vi "Accept Multiple.vi"(8 "error in (no error)":errorcluster, 9 "Number":i32, 10 "Accepted Runes":string, 11 "JSON Lexer in":refnum<class "JSON Lexer.lvclass">) -> (0 "error out":errorcluster, 1 "EOF":bool, 2 "Accepted?":bool, 3 "JSON Lexer out":refnum<class "JSON Lexer.lvclass">)   [LabVIEW 2013, in "JKI JSON Serialization.lvlib" / "JSON Lexer.lvclass"]
uses:
  JSON Lexer.lvclass
  JSON Lexer.lvclass/JSON Lexer.ctl
  <vilib>/addons/_JKI.lib/Unicode/UTF-8 String/UTF-8 String.lvclass/UTF-8 String.ctl
  <vilib>/addons/_JKI.lib/Unicode/UTF-8 String/Index Rune as UTF-8 Substring.vi
  <vilib>/addons/_JKI.lib/Unicode/UTF-8 String/Next Rune As UTF-8 Substring.vi
  <vilib>/addons/_JKI.lib/Unicode/UTF-8 String/Bytes In Rune.vi
  <vilib>/Utility/error.llb/Error Cluster From Error Code.vi
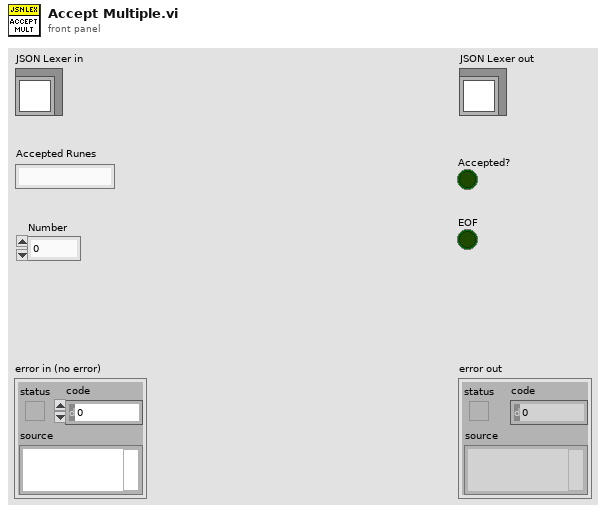
[diagram p1: front panel]
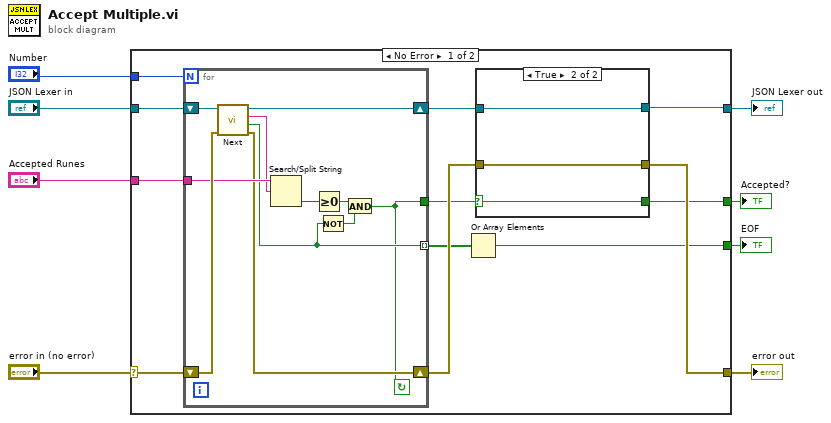
[diagram p0: block diagram]
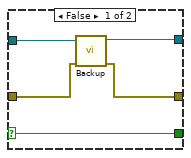
[diagram p2: hidden frame]
diagram:
  n1 = case shown="No Error" "error in (no error)" {
    selector: "error in (no error)" -> [w19 w41]
    tunnel: [w16 w41] -> w7
    tunnel: [w14 w40] -> w5
    tunnel: "JSON Lexer in" -> [w20 w40]
    tunnel: "Accepted Runes" -> [w18 _]
    tunnel: "Number" -> [w13 _]
    tunnel: [w10 _] -> w2
    tunnel: [w9 _] -> w1
    frame No Error {
      n2 = for {
        N: w13 -> [_]
        tunnel: w18 -> [w37]
        shift-right: [w33] -> w15
        shift-left: w20 -> [w39]
        shift-right: [w34] -> w17
        shift-left: w19 -> [w38]
        tunnel: [w29] -> w12
        tunnel: [w30] -> w11 mode=indexing
        stop <- w29 continue-if-true
        n3 = call "Next.vi"("error in (no error)"=w38, "JSON Lexer in"=w39) -> ("error out"=w34:errorcluster, "EOF"=w30:bool, "Rune"=w36:string, "JSON Lexer out"=w33:refnum<class "JSON Lexer.lvclass">)  [unwired: 6 in]
        n4 = Search/Split String(string=w37, search string/char (-)=w36) -> (offset of match=w35:i32)  [unwired: 1 in, 2 out]
        n5 = Greater Or Equal To 0?(x=w35) -> (x >= 0?=w32:bool)
        n6 = Not(x=w30) -> (.not. x?=w31:bool)
        n7 = And(x=w32, y=w31) -> (x .and. y?=w29:bool)
      }
      n8 = Or Array Elements(Boolean array=w11) -> (logical OR=w9:bool)
      n9 = case shown="True" w12 {
        selector: w12 -> [w21 w26]
        tunnel: w17 -> [w25 w27]
        tunnel: [w24 w27] -> w16
        tunnel: w15 -> [w23 w28]
        tunnel: [w22 w28] -> w14
        tunnel: [w21 w26] -> w10
        frame False {
          n10 = call "Backup.vi"("error in (no error)"=w25, "JSON Lexer in"=w23) -> ("error out"=w24:errorcluster, "JSON Lexer out"=w22:refnum<class "JSON Lexer.lvclass">)  [unwired: 8 in]
        }
        frame True {
        }
      }
    }
    frame Error {
    }
  }
  "error out" <- w7
  "JSON Lexer out" <- w5
  "Accepted?" <- w2
  "EOF" <- w1
